vi "20181203_read.vi"() -> ()   [LabVIEW 2017]
uses:
  <vilib>/Utility/file.llb/Write Delimited Spreadsheet (DBL).vi
panel:
  in  "stop":bool
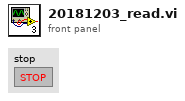
[diagram p1: front panel]
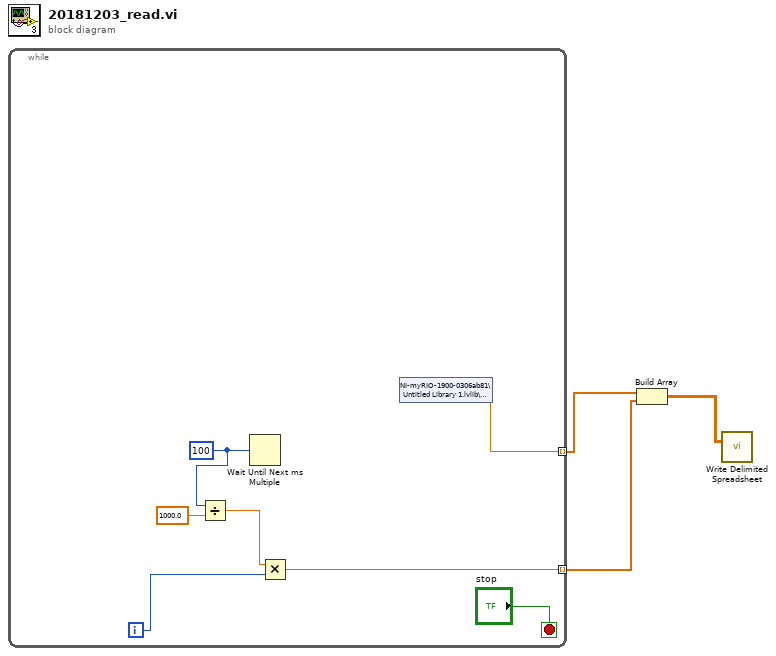
[diagram p0: block diagram]
diagram:
  n1 = while {
    tunnel: [w5] -> w2 mode=indexing
    tunnel: [w4] -> w3 mode=indexing
    i -> [w8]
    stop <- "stop" stop-if-true
    w7 = u32 100 ("millisecond multiple")
    n2 = Divide(x=w7, y=1000.0) -> (x/y=w6:dbl)
    n3 = Wait Until Next ms Multiple(millisecond multiple=w7) -> ()  [unwired: 1 out]
    n4 = Multiply(x=w6, y=w8) -> (x*y=w5:dbl)
    n5 = shared-variable "NI-myRIO-1900-0306ab81\\Untitled Library 1.lvlib\\Variable1"() -> (w4:dbl)  [unwired: 1 in, 1 out]
  }
  n6 = Build Array(w3, w2) -> (w1:dbl[][])
  n7 = call-poly <vilib>:"Write Delimited Spreadsheet.vi"("2D data"=w1) -> ()  [unwired: 13 in, 2 out]
